vi "Log_Calib_Points.vi"(3 "Instrument type":T1=enum."Cross wire velocity", 4 "Root name":string, 5 "Calib file":path=path "/iMac_3 HD/Users/Hong(6%)/calib/XW Ch 1 7_10_02_6") -> ()   [LabVIEW 2020]
uses:
  Controls/Cal_Inst_type.ctl
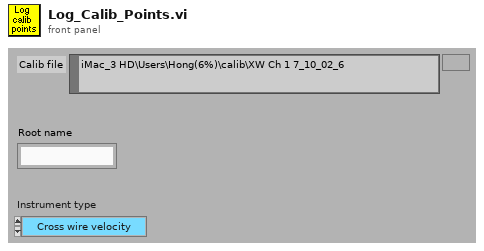
[diagram p1: front panel]
types:
  T1 = typedef "Cal_Inst_type.ctl" = enum16{"Propeller anemometer", "Pressure Transducer", "Hot wire", "Cross wire velocity", "Cross wire angle", "Generic Linear", "Generic Polynomial", "Generic BackPoly", "Fast FID", "Thermocouple", "Cold wire", "Pulsed Wire"}
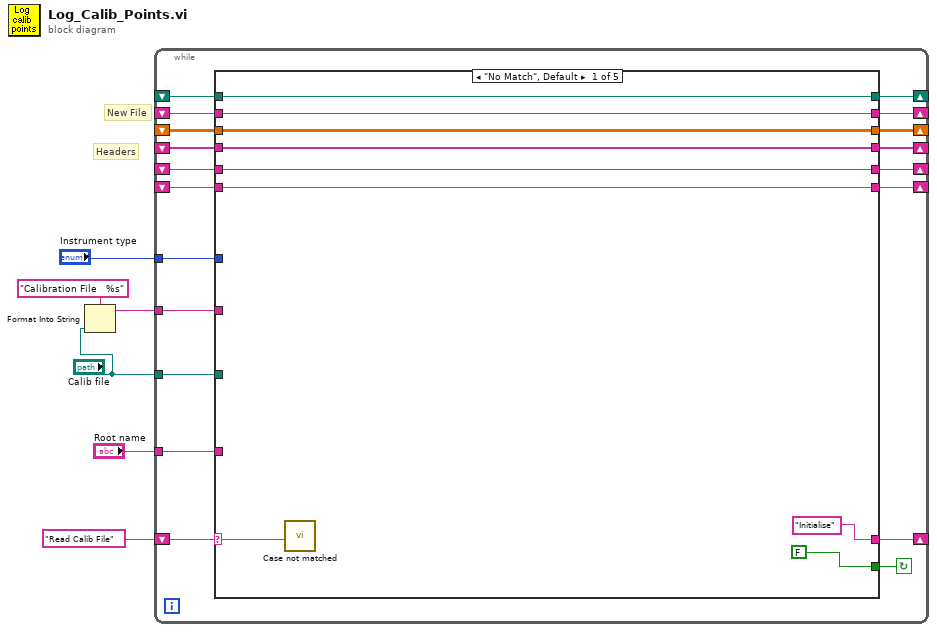
[diagram p0: block diagram]
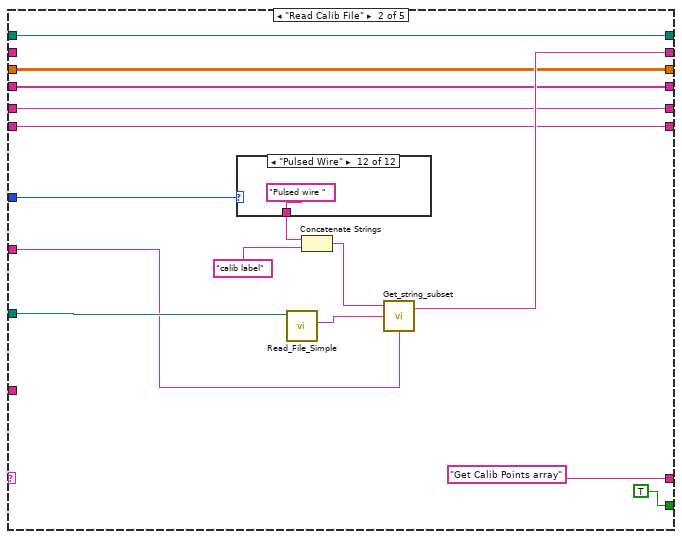
[diagram p2: hidden frame]
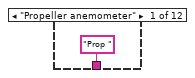
[diagram p3: hidden frame]
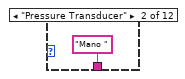
[diagram p4: hidden frame]
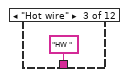
[diagram p5: hidden frame]
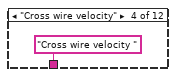
[diagram p6: hidden frame]
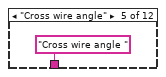
[diagram p7: hidden frame]
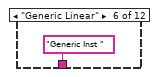
[diagram p8: hidden frame]
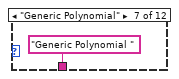
[diagram p9: hidden frame]
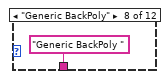
[diagram p10: hidden frame]
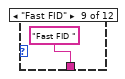
[diagram p11: hidden frame]
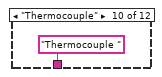
[diagram p12: hidden frame]
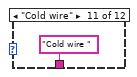
[diagram p13: hidden frame]
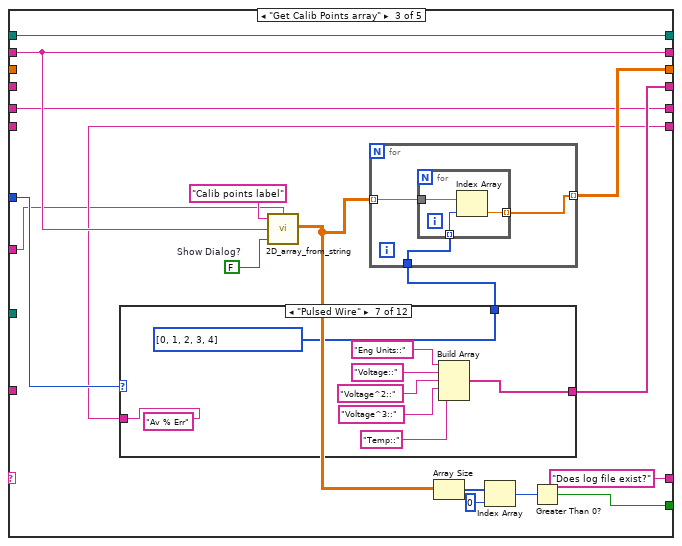
[diagram p14: hidden frame]
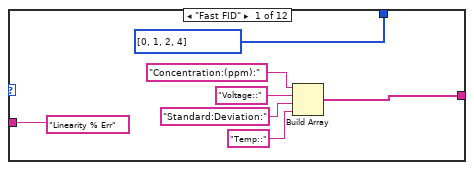
[diagram p15: hidden frame]
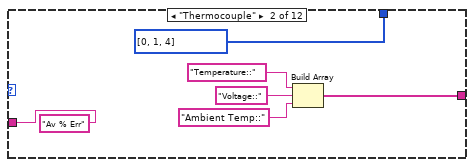
[diagram p16: hidden frame]
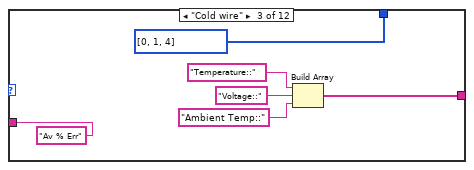
[diagram p17: hidden frame]
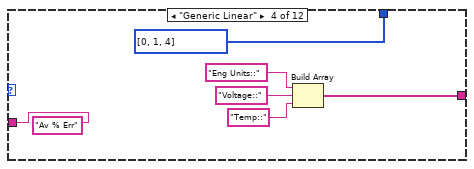
[diagram p18: hidden frame]
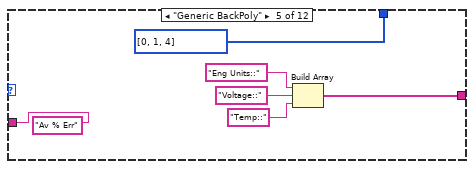
[diagram p19: hidden frame]
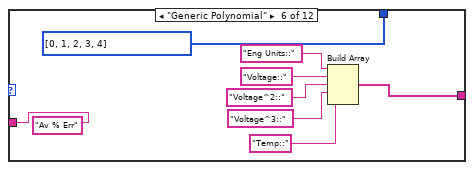
[diagram p20: hidden frame]
diagram:
  # "New File"
  # "Headers"
  n1 = Format Into String(format string="Calibration File   %s", "Calib file") -> (resulting string=w1:string)  [unwired: 2 in, 1 out]
  n2 = while {
    tunnel: "Calib file" -> [w15]
    shift-left: _ -> [w16]
    shift-right: [w17] -> _
    shift-left: _ -> [w18]
    shift-right: [w20] -> _
    tunnel: "Instrument type" -> [w22]
    shift-left: _ -> [w19]
    shift-right: [w21] -> _
    shift-left: "Read Calib File" -> [w23]
    shift-right: [w24] -> _
    tunnel: "Root name" -> [w14]
    shift-right: [w13] -> _
    shift-left: _ -> [w12]
    shift-right: [w11] -> _
    shift-left: _ -> [w10]
    shift-right: [w9] -> _
    shift-left: _ -> [w8]
    tunnel: w1 -> [w7]
    stop <- w25 continue-if-true
    n3 = case shown="\"No Match\", Default" w23 {
      selector: w23 -> [w26 _ _ _ _]
      tunnel: [FALSE TRUE w72 TRUE FALSE] -> w25
      tunnel: ["Initialise" "Get Calib Points array" "Does log file exist?" "Append to log file" "End"] -> w24
      tunnel: w22 -> [_ w45 w76 _ _]
      tunnel: [w32 w44 w71 w171 w202] -> w21
      tunnel: [w31 w39 w65 w174 w215] -> w20
      tunnel: w19 -> [w32 _ w71 w171 w202]
      tunnel: w18 -> [w31 w39 _ w174 w215]
      tunnel: [w30 w43 w68 w175 w212] -> w17
      tunnel: w16 -> [w30 w43 _ w175 w212]
      tunnel: w15 -> [_ w36 _ _ w211]
      tunnel: w14 -> [_ _ _ w167 _]
      tunnel: [w29 w40 w66 w165 w194] -> w13
      tunnel: w12 -> [w29 w40 w66 _ w194]
      tunnel: [w28 w38 w64 w172 w209] -> w11
      tunnel: w10 -> [w28 w38 w64 _ w209]
      tunnel: [w27 w37 w63 w170 w195] -> w9
      tunnel: w8 -> [w27 w37 _ w170 w195]
      tunnel: w7 -> [_ w35 w62 _ _]
      frame "No Match", Default {
        n4 = call "Case not matched.vi"("Case Name not Matched"=w26) -> ()
      }
      frame "Read Calib File" {
        n5 = case shown="\"Pulsed Wire\"" w45 {
          tunnel: ["Prop " "Mano " "HW " "Cross wire velocity " "Cross wire angle " "Generic Inst " "Generic Polynomial " "Generic BackPoly " "Fast FID " "Thermocouple " "Cold wire " "Pulsed wire "] -> w46
          frame "Propeller anemometer" {
          }
          frame "Pressure Transducer" {
          }
          frame "Hot wire" {
          }
          frame "Cross wire velocity" {
          }
          frame "Cross wire angle" {
          }
          frame "Generic Linear" {
          }
          frame "Generic Polynomial" {
          }
          frame "Generic BackPoly" {
          }
          frame "Fast FID" {
          }
          frame "Thermocouple" {
          }
          frame "Cold wire" {
          }
          frame "Pulsed Wire" {
          }
        }
        n6 = call "Read_File_Simple.vi"("Filename"=w36) -> ("string"=w48:string)  [unwired: 2 in, 7 out]
        n7 = Concatenate Strings(w46, "calib label") -> (w42:string)
        n8 = call "Get_string_subset.vi"("String Name"=w35, "String to split"=w48, "File Label"=w42) -> ("Output string"=w44:string)  [unwired: 1 in, 1 out]
      }
      frame "Get Calib Points array" {
        w78 = FALSE  # Show Dialog?
        n9 = case shown="\"Pulsed Wire\"" w76 {
          tunnel: [i32[] [0, 1, 2, 4] i32[] [0, 1, 4] i32[] [0, 1, 4] i32[] [0, 1, 4] i32[] [0, 1, 4] i32[] [0, 1, 2, 3, 4] i32[] [0, 1, 2, 3, 4] i32[] [0, 1, 2, 3, 4] i32[] [0, 1, 2, 4] i32[] [0, 1, 4] i32[] [0, 1, 4] i32[] [0, 1, 4]] -> w70
          tunnel: [w88 w93 w99 w105 w111 w120 w128 w136 w143 w149 w155 w161] -> w65
          tunnel: ["Linearity % Err" "Av % Err" "Av % Err" "Av % Err" "Av % Err" "Av % Err" "Av % Err" "Av % Err" "Av % Err" "Av % Err" "Av % Err" "Av % Err"] -> w63
          frame "Fast FID" {
            n10 = Build Array("Concentration:(ppm):" ("Substring"), "Voltage::" ("Substring"), "Standard:Deviation:" ("Substring"), "Temp::" ("Substring")) -> (w88:string[])
          }
          frame "Thermocouple" {
            n11 = Build Array("Temperature::" ("Substring"), "Voltage::" ("Substring"), "Ambient Temp::" ("Substring")) -> (w93:string[])
          }
          frame "Cold wire" {
            n12 = Build Array("Temperature::" ("Substring"), "Voltage::" ("Substring"), "Ambient Temp::" ("Substring")) -> (w99:string[])
          }
          frame "Generic Linear" {
            n13 = Build Array("Eng Units::" ("Substring"), "Voltage::" ("Substring"), "Temp::" ("Substring")) -> (w105:string[])
          }
          frame "Generic BackPoly" {
            n14 = Build Array("Eng Units::" ("Substring"), "Voltage::" ("Substring"), "Temp::" ("Substring")) -> (w111:string[])
          }
          frame "Generic Polynomial" {
            n15 = Build Array("Eng Units::" ("Substring"), "Voltage::" ("Substring"), "Voltage^2::" ("Substring"), "Voltage^3::" ("Substring"), "Temp::" ("Substring")) -> (w120:string[])
          }
          frame "Pulsed Wire" {
            n16 = Build Array("Eng Units::" ("Substring"), "Voltage::" ("Substring"), "Voltage^2::" ("Substring"), "Voltage^3::" ("Substring"), "Temp::" ("Substring")) -> (w128:string[])
          }
          frame "Cross wire angle" {
            n17 = Build Array("Angle:(degrees):" ("Substring"), "HW1 Voltage::" ("Substring"), "HW2 Voltage::" ("Substring"), "Ref velocity", "Temp::" ("Substring")) -> (w136:string[])
          }
          frame "Cross wire velocity" {
            n18 = Build Array("Velocity::" ("Substring"), "HW1 Voltage::" ("Substring"), "HW2 Voltage::" ("Substring"), "Temp::" ("Substring")) -> (w143:string[])
          }
          frame "Hot wire" {
            n19 = Build Array("Velocity::" ("Substring"), "HW Voltage::" ("Substring"), "Temp::" ("Substring")) -> (w149:string[])
          }
          frame "Propeller anemometer" {
            n20 = Build Array("Velocity::" ("Substring"), "Voltage::" ("Substring"), "Temp::" ("Substring")) -> (w155:string[])
          }
          frame "Pressure Transducer" {
            n21 = Build Array("Pressure::" ("Substring"), "Voltage::" ("Substring"), "Temp::" ("Substring")) -> (w161:string[])
          }
        }
        n22 = call "2D_array_from_string.vi"("String Name"=w62, "Show Dialog?"=w78, "Input string"=w71, "Array title"="Calib points label") -> ("2D data array"=w69:dbl[][])
        n23 = for {
          tunnel: w70 -> [w81]
          tunnel: w69 -> [w80] mode=indexing
          tunnel: [w79] -> w68 mode=indexing
          n24 = for {
            tunnel: w81 -> [w84] mode=indexing
            tunnel: w80 -> [w83]
            tunnel: [w82] -> w79 mode=indexing
            n25 = Index Array(array=w83, index=w84) -> (element=w82:dbl)
          }
        }
        n26 = Array Size(array=w69) -> (size(s)=w75:i32[])
        n27 = Index Array(array=w75, index=0 ("Index")) -> (element=w73:i32)
        n28 = Greater Than 0?(x=w73) -> (x > 0?=w72:bool)
      }
      frame "Does log file exist?" {
        n29 = call "Remove_underscores_at_ends.vi"("String in"=w167) -> ("String out"=w168:string)
        n30 = call "Create_Error_log_folders.vi"("Log Filename"=w168, "Log Folder"="Calib_Points") -> ("Local Log File"=w165:path)  [unwired: 4 in, 1 out]
        n31 = call "Does_file_exist_(simple).vi"("Pathname"=w165) -> ("exists?"=w166:bool)
        n32 = case shown="False" w166 {
          tunnel: w174 -> [w187 _]
          tunnel: [w188 ""] -> w172
          tunnel: w170 -> [w181 _]
          frame False {
            n33 = Concatenate Strings(w181, "::" ("string")) -> (w179:string)
            n34 = Build Array (concatenate)("Date::" ("Substring"), "Time::" ("Substring"), "Seconds:Since:1904" ("Substring"), "Calib:filename:" ("Substring"), w187, w179, "Drift:%:", "Drift:Interval:Minutes") -> (w186:string[])
            n35 = call "Ch_names_to_rows.vi"("Channel Names"=w186) -> ("3 Row names"=w189:string[][])
            n36 = Array To Spreadsheet String(array=w189, 3:"%s" ("format string")) -> (spreadsheet string=w188:string)  [unwired: 1 out]
          }
          frame True {
          }
        }
        n37 = call "Remember_Results_Files.vi"("Filename to Remember"=w165) -> ()  [unwired: 1 out]
      }
      frame "Append to log file" {
        w192 = TRUE  # append to file? (new file:F)
        n38 = call "Get_Characters_from_string.vi"("Input string"=w202, "Variable name"=w195) -> ("Value"=w201:string)  [unwired: 1 in, 1 out]
        n39 = Strip Path(path=w211) -> (name=w198:string)  [unwired: 1 out]
        n40 = Concatenate Strings(w198, "_Drift_Place_Holder" ("Substring")) -> (w197:string)
        n41 = call "Get_Characters_from_string.vi"("Input string"=w202, "Variable name"="Time") -> ("Value"=w204:string)  [unwired: 1 in, 1 out]
        n42 = call "Get_Characters_from_string.vi"("Input string"=w202, "Variable name"="Seconds since 1/1/04") -> ("Value"=w203:string)  [unwired: 1 in, 1 out]
        n43 = call "Get_Characters_from_string.vi"("Input string"=w202, "Variable name"="Date") -> ("Value"=w205:string)  [unwired: 1 in, 1 out]
        n44 = Concatenate Strings(w198, "_Interval_Place_Holder" ("Substring")) -> (w196:string)
        n45 = for {
          tunnel: w212 -> [w227] mode=indexing
          tunnel: w198 -> [w221]
          tunnel: [w225] -> w210 mode=indexing
          tunnel: w205 -> [w224]
          tunnel: w204 -> [w223]
          tunnel: w203 -> [w222]
          tunnel: w201 -> [w220]
          tunnel: w197 -> [w219]
          tunnel: w196 -> [w218]
          n46 = Number To Exponential String(number=w227, precision (6)=i16 10) -> (E-format string=w226:string[])  [unwired: 2 out]
          n47 = Build Array (concatenate)(w224, w223, w222, w221, w226, w220, w219, w218) -> (w225:string[])
        }
        n48 = Array To Spreadsheet String(array=w210, 3:"%s" ("format string")) -> (spreadsheet string=w216:string)  [unwired: 1 out]
        n49 = Concatenate Strings(w209, w216) -> (w193:string)
        n50 = call "Write_File_Simple.vi"("append to file? (new file:F)"=w192, "character string"=w193, "file path"=w194) -> ()  [unwired: 2 out]
      }
    }
  }
